vi "keccak.fpga.top.vi"   [LabVIEW 2021]
uses:
  Users/johns/OneDrive/Documents/LabVIEW Data/Untitled Project 2/CLIP/Keccak.Variables.ctl
  Users/johns/OneDrive/Documents/LabVIEW Data/Untitled Project 2/CLIP/Keccak.States.ctl
  <vilib>/Platform/TimedLoop/XDataNode/timing_clust.ctl
  <vilib>/Platform/TimedLoop/XDataNode/nitl_modes.ctl
  <vilib>/Platform/TimedLoop/XDataNode/wakeup.ctl
  <vilib>/rvi/Emulation/niFpgaSctlEmulationGetInTimedLoop.vi
  <vilib>/rvi/Emulation/niFpgaEmulationReportErrorSimple.vi
  <vilib>/rvi/Emulation/niFpgaGetClockAttributes.vi
  <vilib>/rvi/Emulation/niFpgaCriticalErrorInLSC.vi
  <vilib>/rvi/interface/RandomDataEmulation/niFpgaRandomDataHandleErrors.vi
  <vilib>/platform/TimedLoop/XDataNode/XDataNode.xnode
  <vilib>/rvi/DataTransferAndStorage/Container/XNode/niFpgaContainer.xnode
  <vilib>/rvi/interface/RandomDataEmulation/nirviRandomDataFpgaReadWriteTemplate.vi
  <vilib>/Platform/TimedLoop/XDataNode/XDNodeRunTimeDep.lvlib
types:
  T1 = typedef "Keccak.Variables.ctl" = cluster{"hash.input_size":u16, "hash.bits":u16, "state.next":T2, "state.after_next":T2, "read.i":u16, "read.block_i":u16, "hash.block_words":u16, "hash.block_size":u16, "keccak.i":u16, "state[25]":u64[], "HT_PARMS.Valid":bool, "HT_PARMS.Data":u64, "Read.HT_PARMS":bool, "HT_DATA.Valid":bool, "HT_DATA.Data":u64, "Read.HT_DATA":bool, "TH_RESULTS.Valid":bool, "TH_RESULTS.Data":u64, "TH_RESULTS.Ready":bool}
  T2 = typedef "Keccak.States.ctl" = enum8{"Wait.for.Start", "Read.Blocks", "Read.Remainder", "Keccak", "Send.Result"}
  T3 = typedef "XDNodeRunTimeDep.lvlib/timing_clust.ctl" = cluster{"Expected End [f-1]":u64, "Actual End [f-1]":u64, "Finished Late? [f-1]":bool, "Expected End [i-1]":u64, "Actual End [i-1]":u64, "Finished Late? [i-1]":bool, "Expected Start [i]":u64, "Actual Start [i]":u64, "Expected Start [f]":u64, "Actual Start [f]":u64, "Source Name":string, "Structure Name":string, "Period":i64, "Deadline":i64, "Offset":i64, "Start":i64, "Priority":i32, "Timeout":i32, "Mode":T4, "Wakeup Reason":T5, "Error":errorcluster, "Source Type":string, "Secondary Source Type":string, "Global End Time":u64, "Global Start Time":u64, "Frame Duration":u64, "Iteration Duration":u64, "Assigned CPU":i32, "I/O Scan Engine Mode":u32}
  T4 = typedef "XDNodeRunTimeDep.lvlib/nitl_modes.ctl" = enum32{"No Change", "Process missed periods, maintain original phase", "Discard missed periods, maintain original phase", "Process missed periods, ignore original phase", "Discard missed periods, ignore original phase"}
  T5 = typedef "XDNodeRunTimeDep.lvlib/wakeup.ctl" = enum32{"Normal", "Aborted", "Asynchronous wakeup", "Timing source error", "Timed loop error", "Timeout"}
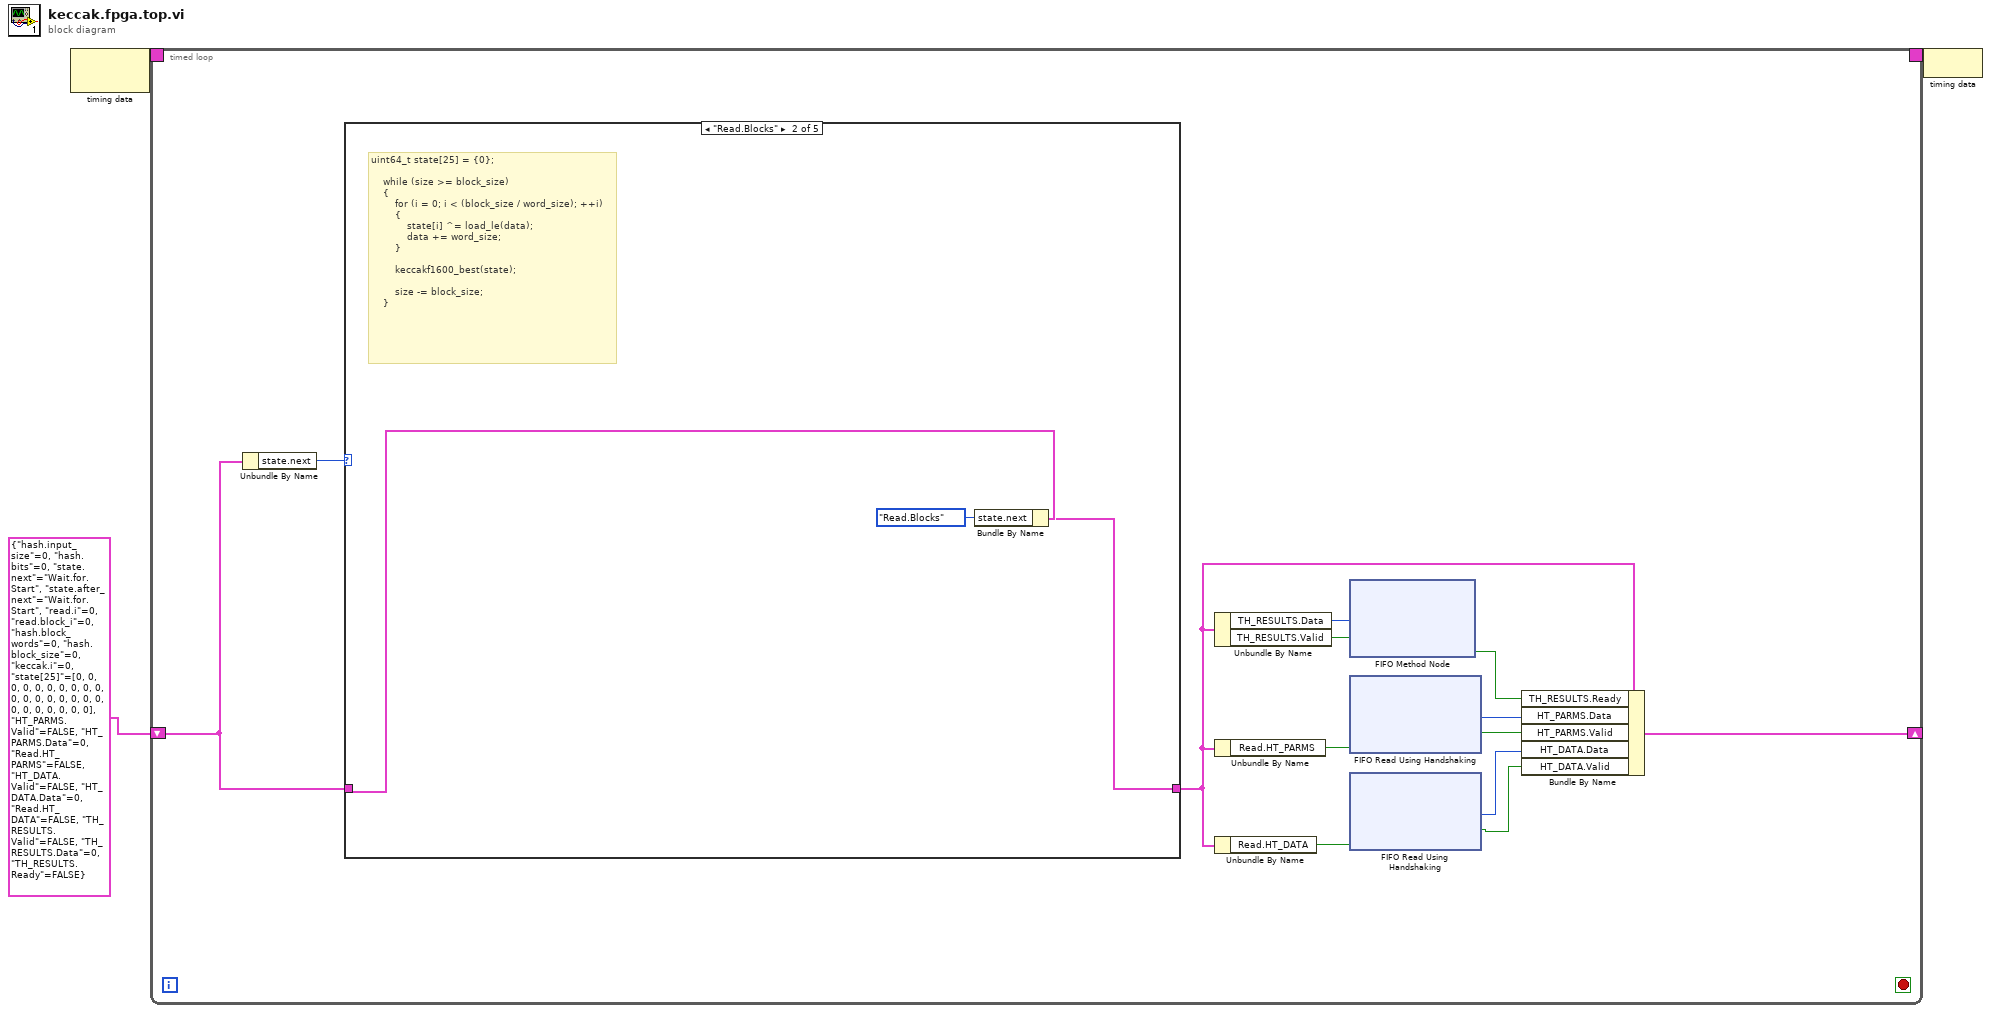
[diagram p0: block diagram]
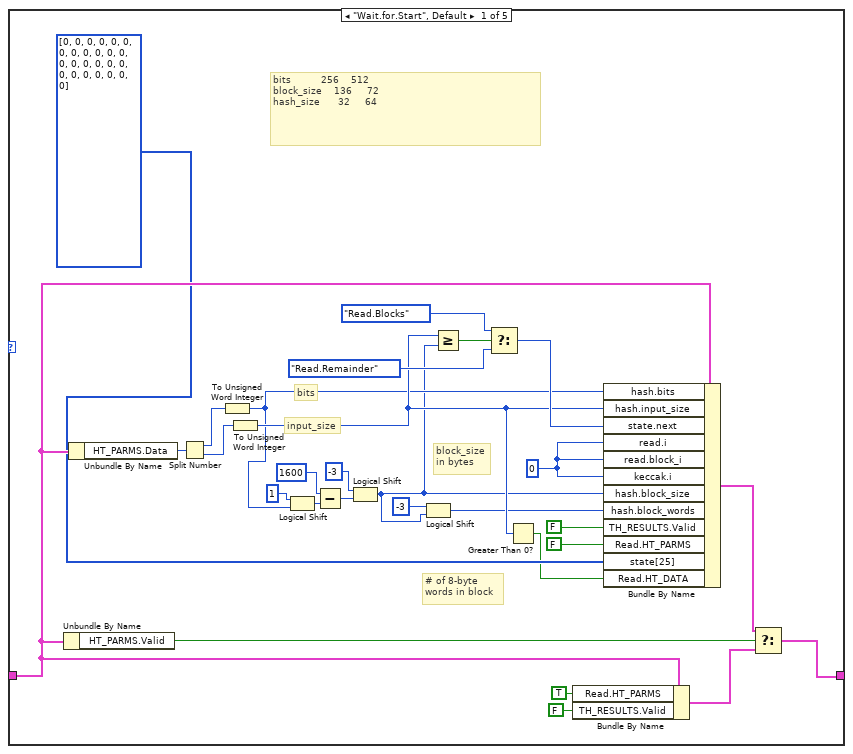
[diagram p2: hidden frame]
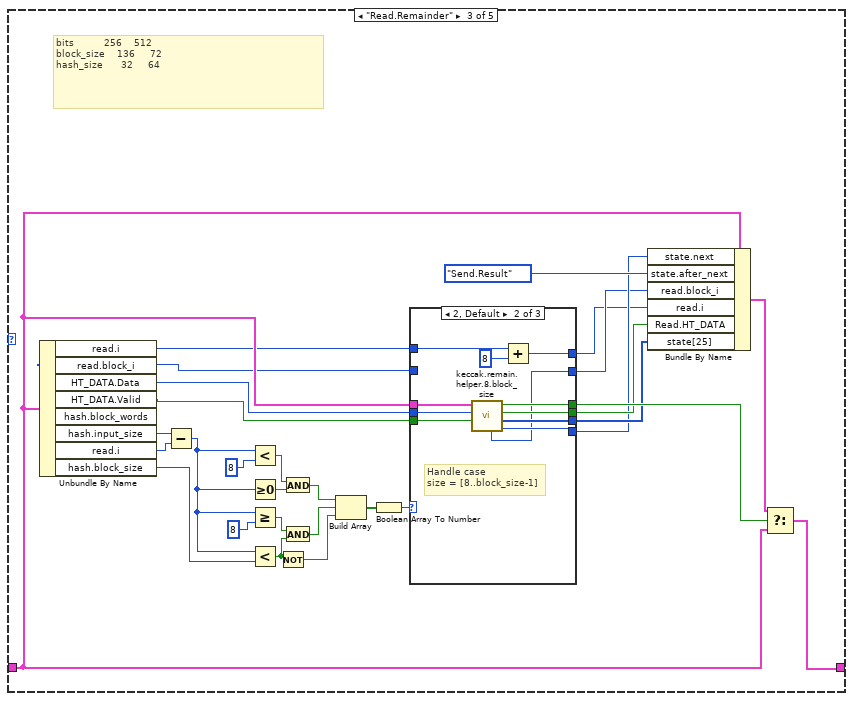
[diagram p3: hidden frame]
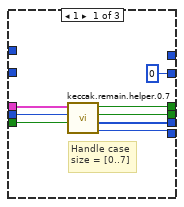
[diagram p4: hidden frame]
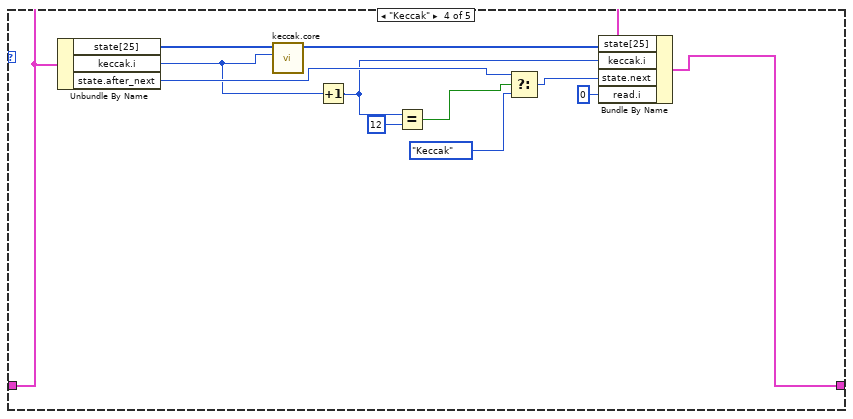
[diagram p6: hidden frame]
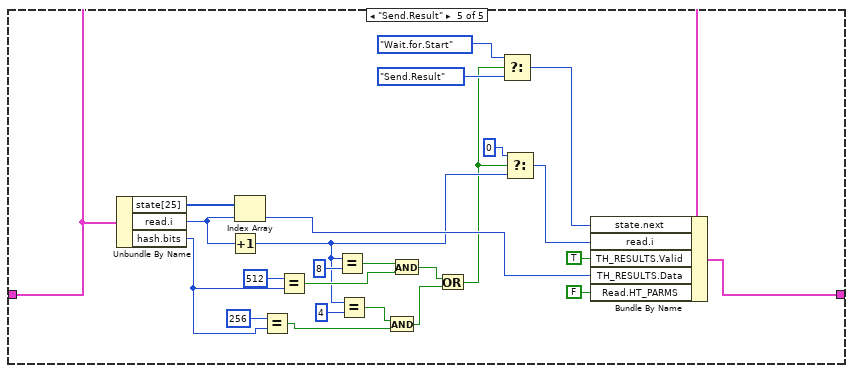
[diagram p7: hidden frame]
diagram:
  n1 = node-c288() -> (w2:T3)  [unwired: 1 in]
  n2 = timed-loop {
    timing: w2 -> [_]
    timing-out: [_] -> w1
    shift-right: [w8] -> _
    shift-left: T1 {"hash.input_size"=0, "hash.bits"=0, "state.next"=enum."Wait.for.Start", "state.after_next"=enum."Wait.for.Start", "read.i"=0, "read.block_i"=0, "hash.block_words"=0, "hash.block_size"=0, "keccak.i"=0, "state[25]"=[0, 0, 0, 0, 0, 0, 0, 0, 0, 0, 0, 0, 0, 0, 0, 0, 0, 0, 0, 0, 0, 0, 0, 0, 0], "HT_PARMS.Valid"=FALSE, "HT_PARMS.Data"=0, "Read.HT_PARMS"=FALSE, "HT_DATA.Valid"=FALSE, "HT_DATA.Data"=0, "Read.HT_DATA"=FALSE, "TH_RESULTS.Valid"=FALSE, "TH_RESULTS.Data"=0, "TH_RESULTS.Ready"=FALSE} ("Variables") -> [w15]
    stop <- _ stop-if-true
    n3 = Unbundle By Name(w15) -> ("state.next"=w16:T2)
    n4 = case shown="\"Read.Blocks\"" w16 {
      tunnel: [w41 w47 w74 w106 w133] -> w7
      tunnel: w15 -> [w36 w48 w69 w107 w132]
      frame "Wait.for.Start", Default {
        w26 = u16 0 ("read.i")
        # "# of 8-byte\nwords in block"
        # "block_size\nin bytes"
        # "bits"
        # "input_size"
        # "bits          256    512\nblock_size    136     72\nhash_size      32     64"
        n5 = Unbundle By Name(w36) -> ("HT_PARMS.Valid"=w40:bool)
        n6 = Unbundle By Name(w36) -> ("HT_PARMS.Data"=w45:u64)
        n7 = Split Number(x=w45) -> (hi(x)=w44:u32, lo(x)=w43:u32)
        n8 = To Unsigned Word Integer(number=w44) -> (unsigned 16bit integer=w18:u16)
        n9 = To Unsigned Word Integer(number=w43) -> (unsigned 16bit integer=w28:u16)
        n10 = Logical Shift(y=i16 1, x=w18) -> (x << y=w23:u16)
        n11 = Subtract(x=u16 1600, y=w23) -> (x-y=w22:u16)
        n12 = Logical Shift(y=i16 -3, x=w22) -> (x << y=w17:u16)
        n13 = Logical Shift(y=i16 -3, x=w17) -> (x << y=w19:u16)
        n14 = Greater Or Equal?(x=w28, y=w17) -> (x >= y?=w32:bool)
        n15 = Select(t=Keccak.States."Read.Blocks" ("state.next"), s=w32, f=Keccak.States."Read.Remainder" ("state.next")) -> (s? t:f=w30:T2)
        n16 = Greater Than 0?(x=w28) -> (x > 0?=w27:bool)
        n17 = Bundle By Name(cluster=w36, "Read.HT_PARMS"=TRUE, "TH_RESULTS.Valid"=FALSE) -> (w37:T1)
        n18 = Bundle By Name(cluster=w36, "hash.bits"=w18, "hash.input_size"=w28, "state.next"=w30, "read.i"=w26, "read.block_i"=w26, "keccak.i"=w26, "hash.block_size"=w17, "hash.block_words"=w19, "TH_RESULTS.Valid"=FALSE, "Read.HT_PARMS"=FALSE, "state[25]"=u64[] [0, 0, 0, 0, 0, 0, 0, 0, 0, 0, 0, 0, 0, 0, 0, 0, 0, 0, 0, 0, 0, 0, 0, 0, 0] ("state[24]"), "Read.HT_DATA"=w27) -> (w42:T1)
        n19 = Select(t=w42, s=w40, f=w37) -> (s? t:f=w41:T1)
      }
      frame "Read.Blocks" {
        # "uint64_t state[25] = {0};\n\n    while (size >= block_size)\n    {\n        for (i = 0; i < (block_size / word_size); ++i)\n        {\n            state[i] ^= load_le(data);\n            data += word_size;\n        }\n\n        keccakf1600_best(state);\n\n        size -= block_size;\n    }"
        n20 = Bundle By Name(cluster=w48, "state.next"=Keccak.States."Read.Blocks") -> (w47:T1)
      }
      frame "Read.Remainder" {
        # "bits          256    512\nblock_size    136     72\nhash_size      32     64"
        n21 = Unbundle By Name(w69) -> ("read.i"=w49:u16, "read.block_i"=w52:u16, "HT_DATA.Data"=w68:u64, "HT_DATA.Valid"=w67:bool, "hash.input_size"=w73:u16, "read.i"=w77:u16, "hash.block_size"=w56:u16)  [unwired: 1 out]
        n22 = Subtract(x=w73, y=w77) -> (x-y=w57:u16)
        n23 = Less?(x=w57, y=u16 8) -> (x < y?=w65:bool)
        n24 = Greater Or Equal To 0?(x=w57) -> (x >= 0?=w66:bool)
        n25 = Greater Or Equal?(x=w57, y=u16 8) -> (x >= y?=w60:bool)
        n26 = Less?(x=w57, y=w56) -> (x < y?=w55:bool)
        n27 = Not(x=w55) -> (.not. x?=w54:bool)
        n28 = And(x=w65, y=w66) -> (x .and. y?=w62:bool)
        n29 = And(x=w60, y=w55) -> (x .and. y?=w59:bool)
        n30 = Build Array(w62, w59, w54) -> (w63:bool[])
        n31 = Boolean Array To Number(Boolean array=w63) -> (number=w61:u8)
        n32 = case shown="2, Default" w61 {
          tunnel: [w85 w92 _] -> w72
          tunnel: [w84 w93 _] -> w71
          tunnel: [w83 w91 _] -> w70
          tunnel: w69 -> [w82 w96 _]
          tunnel: w68 -> [w81 w95 _]
          tunnel: w67 -> [w80 w94 _]
          tunnel: [w79 w87 _] -> w53
          tunnel: w52 -> [_ _ _]
          tunnel: [u16 0 w86 _] -> w51
          tunnel: [_ w89 _] -> w50
          tunnel: w49 -> [_ w88 _]
          frame 1 {
            # "Handle case\nsize = [0..7]"
            n33 = call "keccak.remain.helper.0.7.vi"("HT_DATA.Valid"=w80, "HT_DATA.Data"=w81, "Variables"=w82) -> ("state.next"=w79:T2, "state[25] out"=w83:u64[], "Continue?"=w84:bool, "Valid"=w85:bool)  [unwired: 5 in]
          }
          frame 2, Default {
            # "Handle case\nsize = [8..block_size-1]"
            n34 = call "keccak.remain.helper.8.block_size.vi"("HT_DATA.Valid"=w94, "HT_DATA.Data"=w95, "Variables"=w96) -> ("state.next"=w87:T2, "state[25] out"=w91:u64[], "Continue?"=w93:bool, "Valid"=w92:bool, "read.block_i"=w86:u16)  [unwired: 4 in]
            n35 = Add(x=w88, y=u16 8) -> (x+y=w89:u16)
          }
          frame 4 {
          }
        }
        n36 = Bundle By Name(cluster=w69, "state.next"=w53, "state.after_next"=Keccak.States."Send.Result" ("state.next"), "read.block_i"=w51, "read.i"=w50, "Read.HT_DATA"=w71, "state[25]"=w70) -> (w75:T1)
        n37 = Select(t=w75, s=w72, f=w69) -> (s? t:f=w74:T1)
      }
      frame "Keccak" {
        n38 = Unbundle By Name(w107) -> ("state[25]"=w108:u64[], "keccak.i"=w97:u16, "state.after_next"=w101:T2)
        n39 = call "keccak.core.vi"("keccak.i"=w97, "state[25]"=w108) -> ("state[25].out"=w105:u64[])  [unwired: 9 in]
        n40 = Increment(x=w97) -> (x+1=w99:u16)
        n41 = Equal?(x=w99, y=u16 12) -> (x = y?=w102:bool)
        n42 = Select(t=w101, s=w102, f=Keccak.States."Keccak" ("state.next")) -> (s? t:f=w100:T2)
        n43 = Bundle By Name(cluster=w107, "state[25]"=w105, "keccak.i"=w99, "state.next"=w100, "read.i"=u16 0) -> (w106:T1)
      }
      frame "Send.Result" {
        n44 = Unbundle By Name(w132) -> ("state[25]"=w131:u64[], "read.i"=w130:u16, "hash.bits"=w120:u16)
        n45 = Increment(x=w130) -> (x+1=w113:u16)
        n46 = Index Array(array=w131, index=w130) -> (element=w121:u64)
        n47 = Equal?(x=u16 256, y=w120) -> (x = y?=w117:bool)
        n48 = Equal?(x=u16 512, y=w120) -> (x = y?=w126:bool)
        n49 = Equal?(x=w113, y=u16 8) -> (x = y?=w127:bool)
        n50 = Equal?(x=w113, y=u16 4) -> (x = y?=w116:bool)
        n51 = And(x=w116, y=w117) -> (x .and. y?=w115:bool)
        n52 = And(x=w127, y=w126) -> (x .and. y?=w114:bool)
        n53 = Or(x=w114, y=w115) -> (x .or. y?=w111:bool)
        n54 = Select(t=Keccak.States."Wait.for.Start" ("state.next"), s=w111, f=Keccak.States."Send.Result" ("state.next")) -> (s? t:f=w123:T2)
        n55 = Select(t=u16 0, s=w111, f=w113) -> (s? t:f=w112:u16)
        n56 = Bundle By Name(cluster=w132, "state.next"=w123, "read.i"=w112, "TH_RESULTS.Valid"=TRUE, "TH_RESULTS.Data"=w121, "Read.HT_PARMS"=FALSE) -> (w133:T1)
      }
    }
    n57 = Unbundle By Name(w7) -> ("TH_RESULTS.Data"=w6:u64, "TH_RESULTS.Valid"=w5:bool)
    n58 = Unbundle By Name(w7) -> ("Read.HT_PARMS"=w13:bool)
    n59 = Unbundle By Name(w7) -> ("Read.HT_DATA"=w14:bool)
    n60 = xnode ("FIFO Method Node")("Element"=w6, "Input Valid"=w5) -> ("Ready for Input"=w4:bool)  [unwired: 1 in, 1 out]
    n61 = xnode ("FIFO Read Using Handshaking")("Ready for Output"=w13) -> ("Element"=w11:u64, "Output Valid"=w12:bool)  [unwired: 1 in, 1 out]
    n62 = xnode ("FIFO Read Using Handshaking")("Ready for Output"=w14) -> ("Element"=w9:u64, "Output Valid"=w10:bool)  [unwired: 1 in, 1 out]
    n63 = Bundle By Name(cluster=w7, "TH_RESULTS.Ready"=w4, "HT_PARMS.Data"=w11, "HT_PARMS.Valid"=w12, "HT_DATA.Data"=w9, "HT_DATA.Valid"=w10) -> (w8:T1)
  }
  n64 = node-c288(w1) -> ()
